vi "fancy new vi   test.vi"() -> ()   [LabVIEW 2018]
uses:
  fancy new type.ctl
  <vilib>/event_ctls.llb/eventvkey.ctl
panel:
  in  "control something":T1=enum."mul"
  in  "A":dbl(slide) scale=0.0..10.0
  out "c":dbl
  in  "B":dbl(slide) scale=0.0..10.0
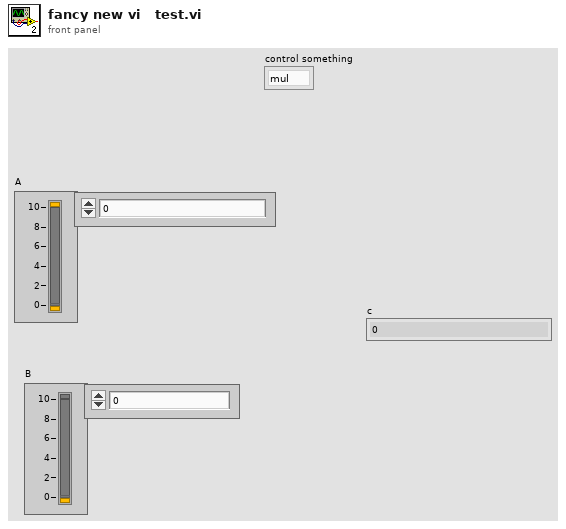
[diagram p1: front panel]
types:
  T1 = typedef "fancy new type.ctl" = enum16{"add", "sub", "mul"}
  T2 = typedef "eventvkey.ctl" = enum16{"ASCII", "Enter", "Return", "Shift", "Ctrl", "Alt", "Cmd", "Opt", "Caps", "NumLock", "Clear", "Break", "Up", "Down", "Left", "Right", "Insert", "Delete", "Home", "End", "PageUp", "PageDown", "Escape", "Help", "Pause", "ScrollLock", "F1", "F2", "F3", "F4", "F5", "F6", "F7", "F8", "F9", "F10", "F11", "F12", "F13", "F14", "F15", "F16", "F17", "F18", "F19", "F20", "F21", "F22", "F23", "F24", "Play", "VolumeUp", "VolumeDown", "Mute", "Two Byte Char"}
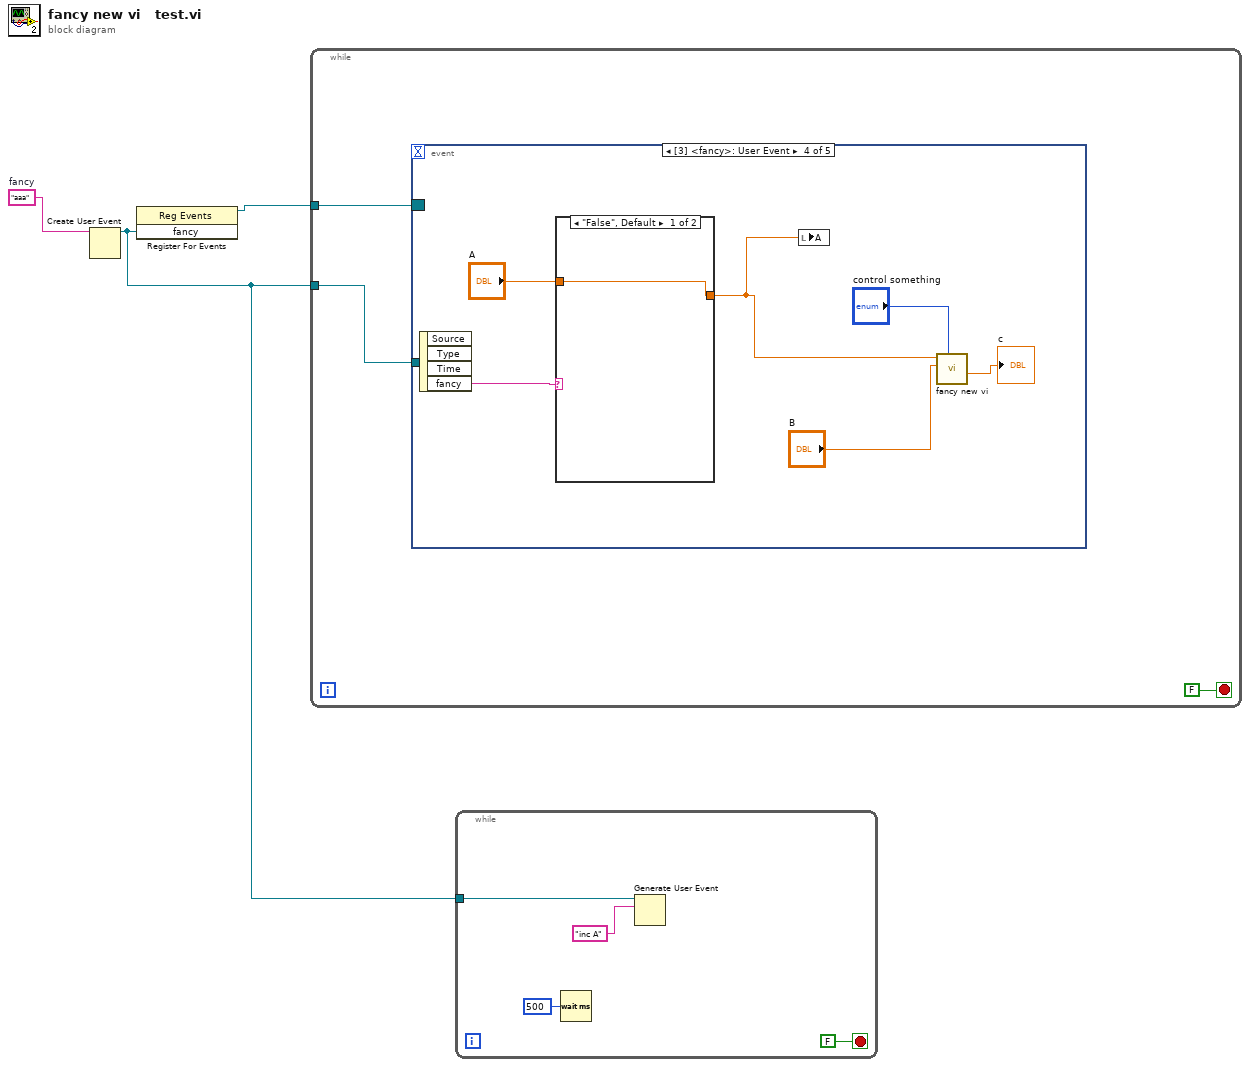
[diagram p0: block diagram]
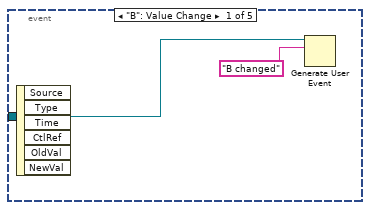
[diagram p2: hidden frame]
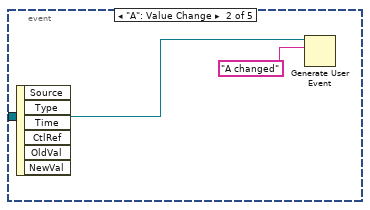
[diagram p3: hidden frame]
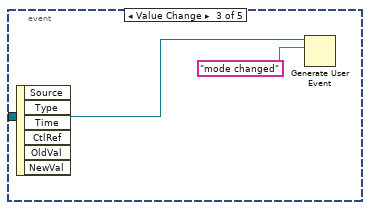
[diagram p4: hidden frame]
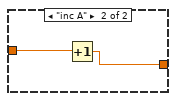
[diagram p5: hidden frame]
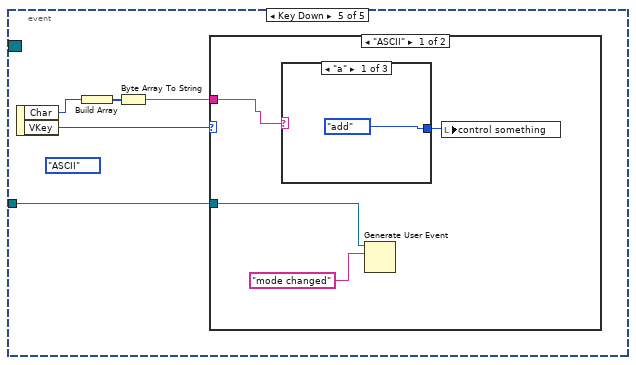
[diagram p6: hidden frame]
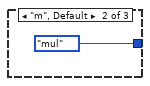
[diagram p7: hidden frame]
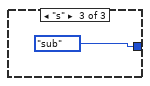
[diagram p8: hidden frame]
diagram:
  w3 = "aaa"  # fancy
  n1 = Create User Event(user event datatype=w3) -> (user event=w1:refnum<user-event>)  [unwired: 1 in, 1 out]
  n2 = register-events(w1) -> (reference out=w2:refnum<event-registration>)  [unwired: 2 in, 1 out]
  n3 = while {
    tunnel: w2 -> [w5]
    tunnel: w1 -> [w4]
    stop <- FALSE stop-if-true
    n4 = event shown="[3] <fancy>: User Event" {
      selector: w5 -> [_ _ _ _ _]
      dyn-events: _ -> [_ _ _ _ _]
      timeout: _ -> [_ _ _ _ _]
      tunnel: w4 -> [w8 w10 w12 _ w22]
      event "B": Value Change {
        n5 = event-data() -> ()  [unwired: 1 in, 6 out]
        n6 = Generate User Event(user event=w8, event data cluster="B changed" ("event data")) -> ()  [unwired: 2 in, 2 out]
      }
      event "A": Value Change {
        n7 = event-data() -> ()  [unwired: 1 in, 6 out]
        n8 = Generate User Event(user event=w10, event data cluster="A changed" ("event data")) -> ()  [unwired: 2 in, 2 out]
      }
      event Value Change {
        n9 = event-data() -> ()  [unwired: 1 in, 6 out]
        n10 = Generate User Event(user event=w12, event data cluster="mode changed" ("event data")) -> ()  [unwired: 2 in, 2 out]
      }
      event User Event {
        n11 = event-data() -> ("fancy"=w18:string)  [unwired: 1 in, 3 out]
        n12 = case shown="\"False\", Default" w18 {
          tunnel: [w19 w20] -> w13
          tunnel: "A" -> [w19 w21]
          frame "False", Default {
          }
          frame "inc A" {
            n13 = Increment(x=w21) -> (x+1=w20:dbl)
          }
        }
        n14 = local write "A"(w13) -> ()
        n15 = call "fancy new vi.vi"("control something"="control something", "b"="B", "a"=w13) -> ("c"=→"c":dbl)  [unwired: 6 in]
      }
      event Key Down {
        (unwired) eventvkey."ASCII" ("VKey")
        n16 = event-data() -> ("Char"=w24:i16, "VKey"=w26:T2)  [unwired: 1 in]
        n17 = Build Array(w24) -> (w25:i16[])
        n18 = Byte Array To String(unsigned byte array=w25) -> (string=w23:string)
        n19 = case shown="\"ASCII\"" w26 {
          tunnel: w23 -> [w30 _]
          tunnel: w22 -> [w28 _]
          frame "ASCII" {
            n20 = case shown="\"a\"" w30 {
              tunnel: [fancy_new_type."add" ("control something") fancy_new_type."mul" ("control something") fancy_new_type."sub" ("control something")] -> w29
              frame "a" {
              }
              frame "m", Default {
              }
              frame "s" {
              }
            }
            n21 = Generate User Event(user event=w28, event data cluster="mode changed" ("event data")) -> ()  [unwired: 2 in, 2 out]
            n22 = local write "control something"(w29) -> ()
          }
          frame "Enter", Default {
          }
        }
      }
    }
  }
  n23 = while {
    tunnel: w1 -> [w35]
    stop <- FALSE stop-if-true
    n24 = Wait (ms)(milliseconds to wait=u32 500) -> ()  [unwired: 1 out]
    n25 = Generate User Event(user event=w35, event data cluster="inc A" ("event data")) -> ()  [unwired: 2 in, 2 out]
  }
